vi "task_configHardware.vi"() -> ()   [LabVIEW 2015]
uses:
  Framework/pdbm_test_route/UsrDefine/TaskFeedbackCmd.ctl
  Framework/pdbm_test_route/UsrDefine/TaskReqst.ctl
  Framework/pdbm_tasks/pdbm_tasks.lvlib
  Framework/pdbm_test_route/pdbm_task_route.lvlib
panel:
  in  "Tab Control":T1(tab)
  in  "CANSensor":cluster{"port":i32, "baud":i32} {"baud" min=0; "port" min=0}
  in  "SensorComm":T2={"Communication"={"Port"=0, "Baud rate"=9600, "Parity check"=enum."Even", "Transmission mode"=enum."RTU", "Time out"=0}, "SensorAddr"={"top_oil_sensor_addr"=0, "bot_oil_sensor_addr"=0, "amb_sensor_addr"=0, "vol_meas_sensor_addr"=0}} {"Communication"."Port" items=["COM1", "COM3"]; "Communication"."Baud rate" items=["1200"=1200, "2400"=2400, "4800"=4800, "9600"=9600, "19200"=19200, "38400"=38400, "57600"=57600, "115200"=115200]}
  in  "MeasComm":T3={"Main CPU"={"Port"=0, "Baud rate"=9600}, "FPGA Port 1"={"Port"=0, "Baud rate"=9600}, "FPGA Port 2"={"Port"=0, "Baud rate"=9600}} {"FPGA Port 2"."Baud rate" items=["1200"=1200, "2400"=2400, "4800"=4800, "9600"=9600, "19200"=19200, "38400"=38400, "57600"=57600, "115200"=115200]; "FPGA Port 2"."Port" items=["COM1", "COM3"]; "FPGA Port 1"."Baud rate" items=["1200"=1200, "2400"=2400, "4800"=4800, "9600"=9600, "19200"=19200, "38400"=38400, "57600"=57600, "115200"=115200]; "FPGA Port 1"."Port" items=["COM1", "COM3"]; "Main CPU"."Baud rate" items=["1200"=1200, "2400"=2400, "4800"=4800, "9600"=9600, "19200"=19200, "38400"=38400, "57600"=57600, "115200"=115200]; "Main CPU"."Port" items=["COM1", "COM3"]}
  in  "PDGen":cluster{"Port":u16, "Baud rate":u32}={"Port"=0, "Baud rate"=9600} {"Baud rate" items=["1200"=1200, "2400"=2400, "4800"=4800, "9600"=9600, "19200"=19200, "38400"=38400, "57600"=57600, "115200"=115200]; "Port" items=["COM1", "COM3"]}
  in  "error in (no error)":errorcluster
  in  "pdbm_task_data":T4
  # "[ms]"
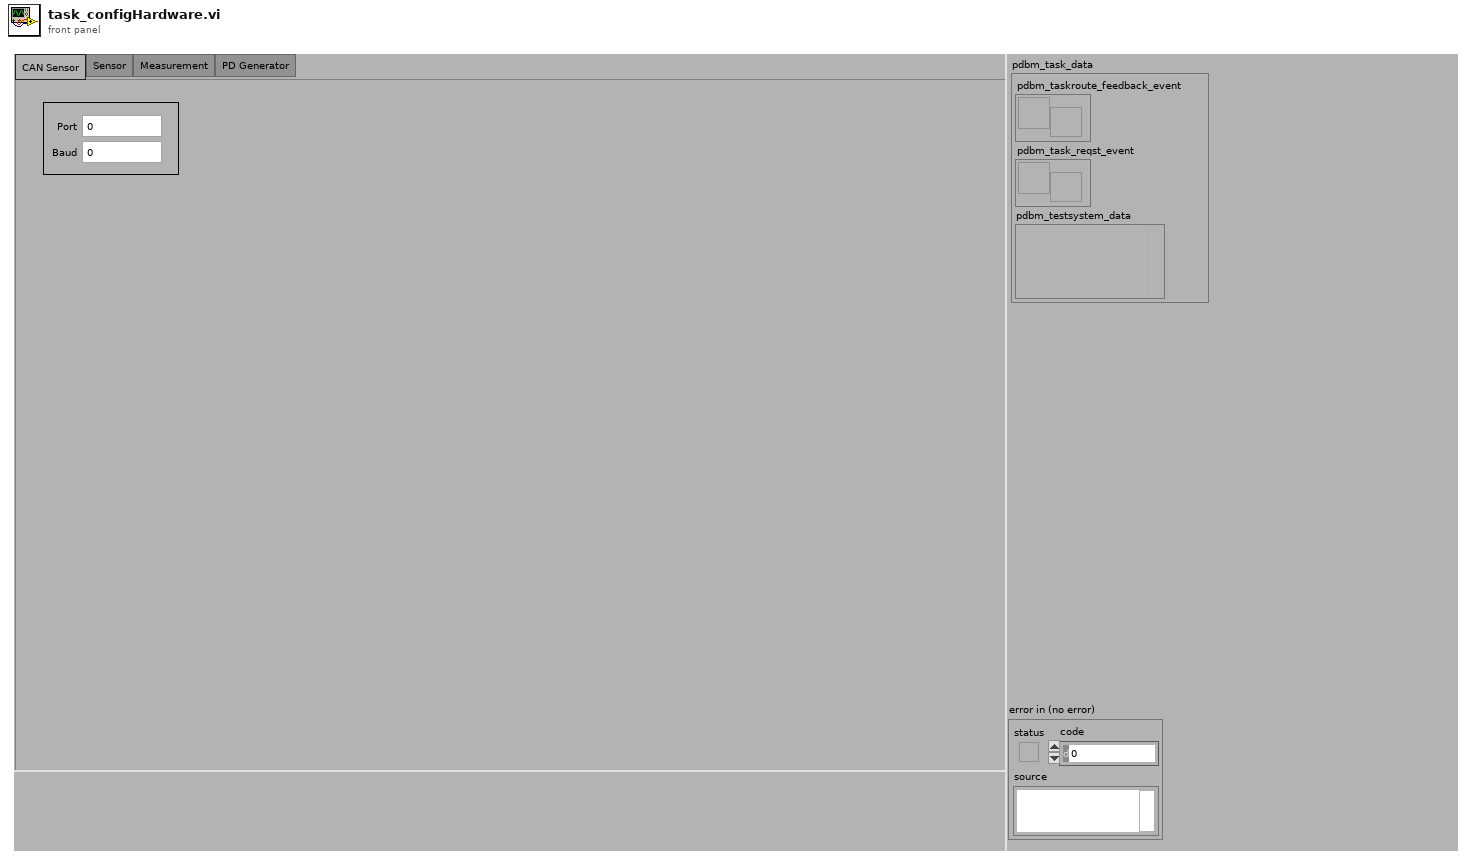
[diagram p1: front panel]
types:
  T1 = enum32{"CAN Sensor", "Sensor", "Measurement", "PD Generator"}
  T2 = cluster{"Communication":cluster{"Port":u16, "Baud rate":u32, "Parity check":enum16{"Odd", "Even", "None"}, "Transmission mode":enum16{"RTU", "ASCII"}, "Time out":u32}, "SensorAddr":cluster{"top_oil_sensor_addr":u8, "bot_oil_sensor_addr":u8, "amb_sensor_addr":u8, "vol_meas_sensor_addr":u8}}
  T3 = cluster{"Main CPU":cluster{"Port":u16, "Baud rate":u32}, "FPGA Port 1":cluster{"Port":u16, "Baud rate":u32}, "FPGA Port 2":cluster{"Port":u16, "Baud rate":u32}}
  T4 = cluster{"pdbm_taskroute_feedback_event":refnum<user-event>, "pdbm_task_reqst_event":refnum<user-event>, "pdbm_testsystem_data":variant}
  T5 = typedef "pdbm_tasks.lvlib/PDBM_TestSystem_Data.ctl" = cluster{"pdbm_general_report_info":refnum<vi>, "pdbm_task_progress":refnum<vi>, "pdbm_TestButton":refnum<vi>}
  T6 = cluster{"pdbm_task_reqst_event":refnum<user-event>, "pdbm_taskroute_feedback_event":refnum<user-event>}
  T7 = typedef "pdbm_tasks.lvlib/TaskRequest.ctl" = cluster{"Command":string, "Variant":variant}
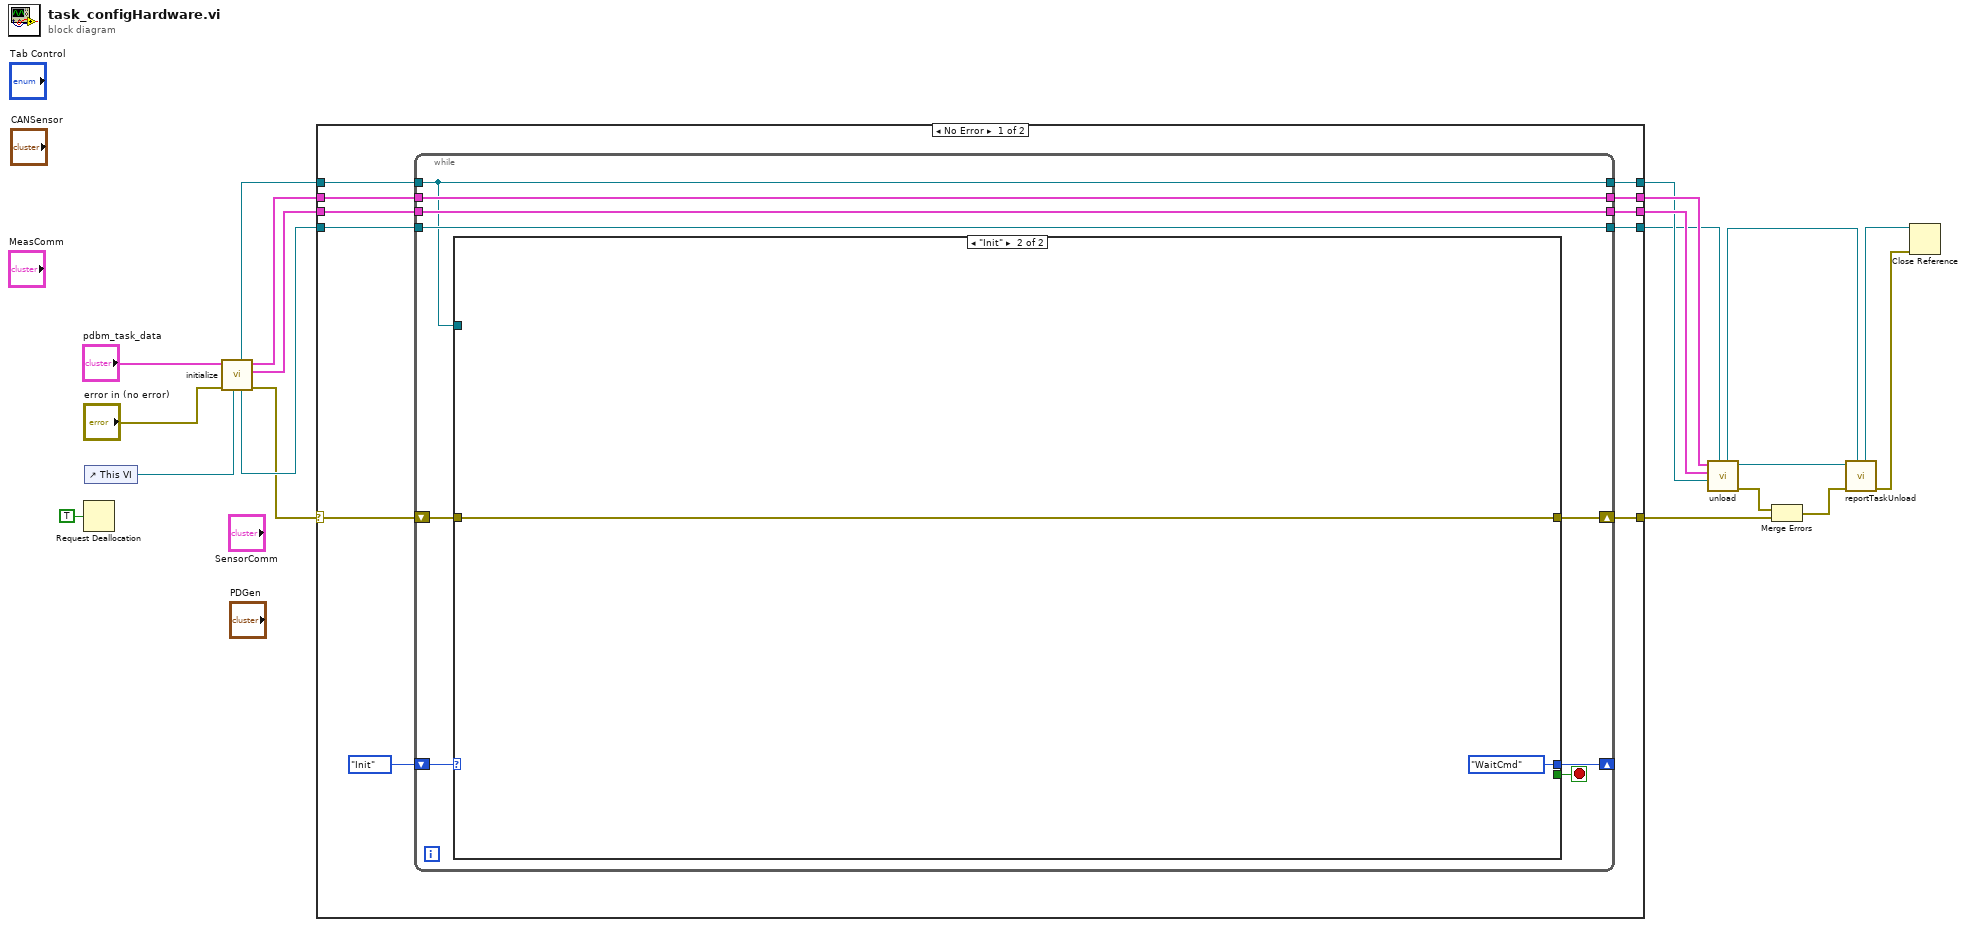
[diagram p0: block diagram]
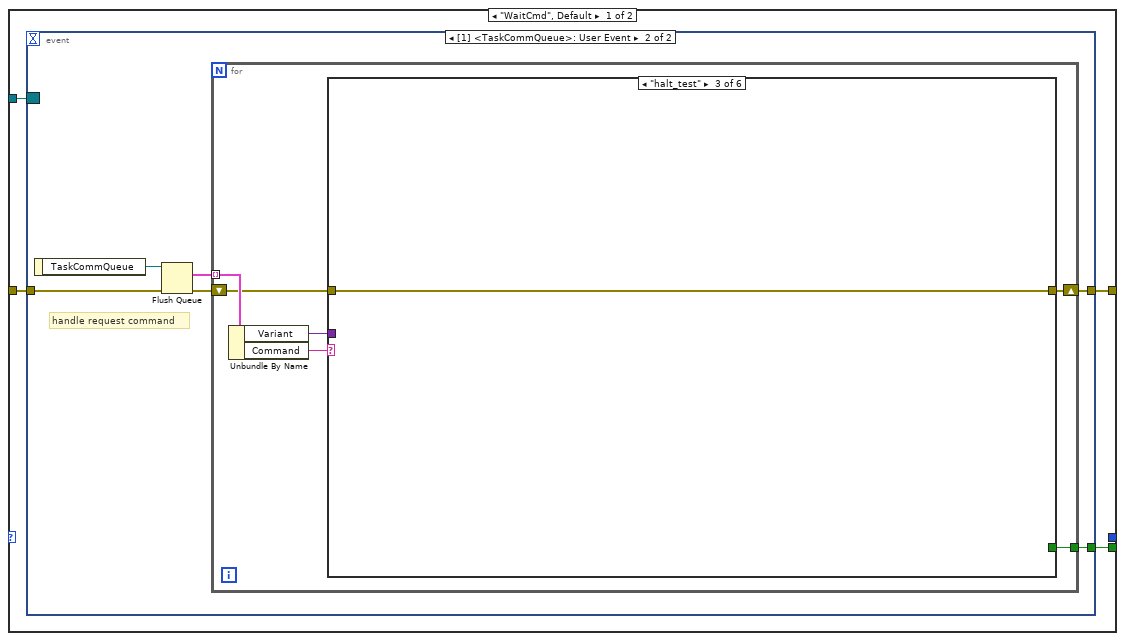
[diagram p2: hidden frame]
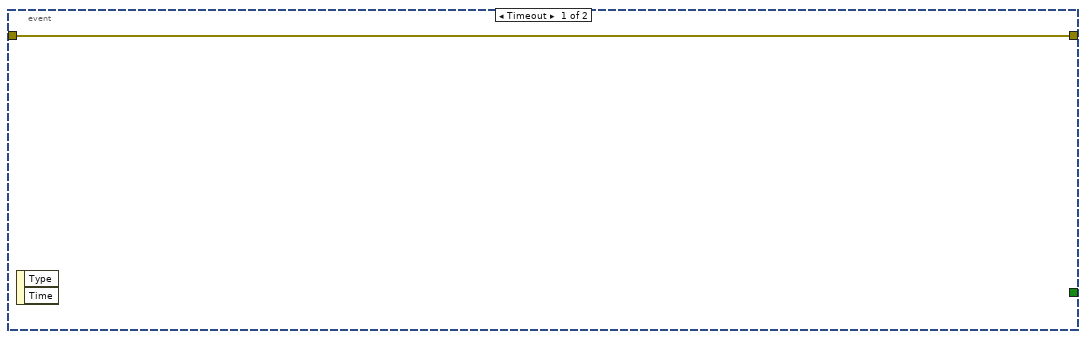
[diagram p3: hidden frame]
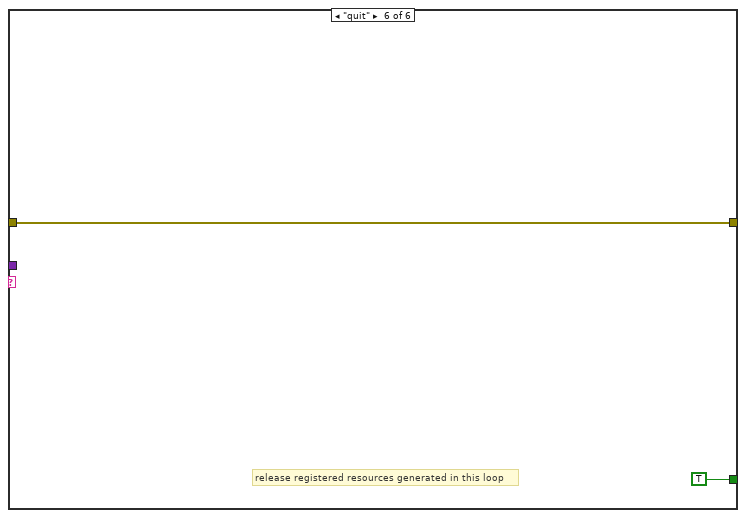
[diagram p8: hidden frame]
diagram:
  n1 = Request Deallocation(TRUE ("flag")) -> ()
  n2 = control-ref of="This VI"() -> (w19:refnum<vi>)
  n3 = call "initialize.vi"("TaskRef in"=w19, "error in"="error in (no error)", "pdbm_task_data"="pdbm_task_data") -> ("error out"=w15:errorcluster, "pdbm_task_data"=w3:T5, "pdbm_task_event"=w16:T6, "TaskRef out"=w17:refnum<vi>, "pdbm_task_reg_reqst_event"=w14:refnum<event-registration>)  [unwired: 4 in]
  n4 = case shown="No Error" w15 {
    selector: w15 -> [w30 w71]
    tunnel: w3 -> [w28 w69]
    tunnel: [w29 w71] -> w10
    tunnel: w17 -> [w23 w68]
    tunnel: w16 -> [w27 w70]
    tunnel: w14 -> [w31 w67]
    tunnel: [w26 w70] -> w13
    tunnel: [w25 w69] -> w12
    tunnel: [w24 w68] -> w2
    tunnel: [w22 w67] -> w11
    frame No Error {
      n5 = while {
        tunnel: w31 -> [w34]
        shift-right: [w39] -> w29
        shift-left: w30 -> [w40]
        tunnel: w23 -> [w35]
        tunnel: w28 -> [w36]
        tunnel: w27 -> [w37]
        tunnel: [w37] -> w26
        tunnel: [w36] -> w25
        tunnel: [w35] -> w24
        tunnel: [w34] -> w22
        shift-right: [w32] -> _
        shift-left: enum16{"WaitCmd", "Init"}."Init" -> [w33]
        stop <- w38 stop-if-true
        n6 = case shown="\"Init\"" w33 {
          tunnel: w40 -> [w44 w65]
          tunnel: [w43 w65] -> w39
          tunnel: [w42 _] -> w38
          tunnel: w34 -> [w41 _]
          tunnel: [_ enum16{"WaitCmd", "Init"}."WaitCmd"] -> w32
          frame "WaitCmd", Default {
            n7 = event shown="[1] <TaskCommQueue>: User Event" {
              selector: w41 -> [_ _]
              dyn-events: _ -> [_ _]
              timeout: _ -> [_ _]
              tunnel: w44 -> [w45 w50]
              tunnel: [w45 w47] -> w43
              tunnel: [_ w46] -> w42
              event Timeout {
                n8 = event-data() -> ()  [unwired: 1 in, 2 out]
              }
              event User Event {
                # "handle request command"
                n9 = event-data() -> ("TaskCommQueue"=w51:refnum<queue>)  [unwired: 1 in]
                n10 = Flush Queue(queue=w51, error in (no error)=w50) -> (remaining elements=w48:T7[], error out=w49:errorcluster)  [unwired: 1 out]
                n11 = for {
                  tunnel: w48 -> [w57] mode=indexing
                  shift-right: [w53] -> w47
                  shift-left: w49 -> [w55]
                  tunnel: [w52] -> w46
                  n12 = Unbundle By Name(w57) -> ("Variant"=w54:variant, "Command"=w56:string)
                  n13 = case shown="\"halt_test\"" w56 {
                    tunnel: w55 -> [w58 w59 w60 w61 w62 w64]
                    tunnel: w54 -> [_ _ _ _ _ _]
                    tunnel: [w58 w59 w60 w61 w62 w64] -> w53
                    tunnel: [_ _ _ _ _ TRUE] -> w52
                    frame "False", Default {
                    }
                    frame "exeTest" {
                    }
                    frame "halt_test" {
                    }
                    frame "stop_test" {
                    }
                    frame "ReInit" {
                      # "ReInitialize your VI"
                    }
                    frame "quit" {
                      # "release registered resources generated in this loop"
                    }
                  }
                }
              }
            }
          }
          frame "Init" {
          }
        }
      }
    }
    frame Error {
    }
  }
  n14 = call "unload.vi"("TaskRef in"=w2, "pdbm_task_reg_reqst_event"=w11, "pdbm_task_data"=w12, "pdbm_task_event"=w13) -> ("error out"=w9:errorcluster, "pdbm_taskroute_feedback_event"=w8:refnum<user-event>, "TaskRef out"=w1:refnum<vi>)  [unwired: 5 in]
  n15 = Merge Errors(w9, w10) -> (w7:errorcluster)
  n16 = call "reportTaskUnload.vi"("TaskRef"=w1, "error in (no error)"=w7, "pdbm_taskroute_feedback_event"=w8) -> ("error out"=w4:errorcluster, "TaskRef out"=w5:refnum<vi>)  [unwired: 6 in, 1 out]
  n17 = Close Reference(reference=w5, error in (no error)=w4) -> ()  [unwired: 1 out]
